vi "OlfactoryStim.vi"() -> ()   [LabVIEW 2014]
uses:
  Stim/Stim.lvclass
  <vilib>/Platform/TimedLoop/XDataNode/timing_clust.ctl
  <vilib>/Platform/TimedLoop/XDataNode/nitl_modes.ctl
  <vilib>/Platform/TimedLoop/XDataNode/wakeup.ctl
  Acquisition/Acquisition.lvclass
  <vilib>/platform/TimedLoop/XDataNode/XDataNode.xnode
  <vilib>/Platform/TimedLoop/XDataNode/XDNodeRunTimeDep.lvlib
panel:
  in  "ITA \nchannel":dbl
  in  "Cardname":string="DevOlf"
  in  "depth(um)":dbl
  in  "notes":string
  in  "filename":string
  out "error out":errorcluster
  in  "Idx":dbl[](array[numeric])
  in  "Stimulus Description":string[](array[string])
  in  "mouse_id":dbl
  out "Trial":dbl
  out "stim queue":i32
  in  "semicolon seperated stimuli":string
  in  "ITI (ms)":dbl=4000.0
  in  "Pulse Dur (ms)":dbl=4000.0
  in  "stop":bool
  out "Stim":bool[](array[boolean])
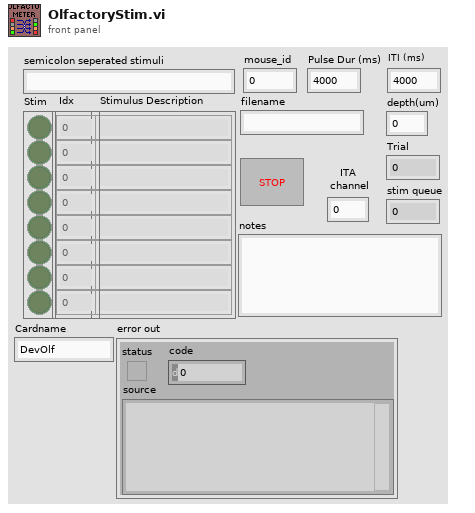
[diagram p1: front panel]
types:
  T1 = typedef "XDNodeRunTimeDep.lvlib/timing_clust.ctl" = cluster{"Expected End [f-1]":u64, "Actual End [f-1]":u64, "Finished Late? [f-1]":bool, "Expected End [i-1]":u64, "Actual End [i-1]":u64, "Finished Late? [i-1]":bool, "Expected Start [i]":u64, "Actual Start [i]":u64, "Expected Start [f]":u64, "Actual Start [f]":u64, "Source Name":string, "Structure Name":string, "Period":i64, "Deadline":i64, "Offset":i64, "Start":i64, "Priority":i32, "Timeout":i32, "Mode":T2, "Wakeup Reason":T3, "Error":errorcluster, "Source Type":string, "Secondary Source Type":string, "Global End Time":u64, "Global Start Time":u64, "Frame Duration":u64, "Iteration Duration":u64, "Assigned CPU":i32, "I/O Scan Engine Mode":u32}
  T2 = typedef "XDNodeRunTimeDep.lvlib/nitl_modes.ctl" = enum32{"No Change", "Process missed periods, maintain original phase", "Discard missed periods, maintain original phase", "Process missed periods, ignore original phase", "Discard missed periods, ignore original phase"}
  T3 = typedef "XDNodeRunTimeDep.lvlib/wakeup.ctl" = enum32{"Normal", "Aborted", "Asynchronous wakeup", "Timing source error", "Timed loop error", "Timeout"}
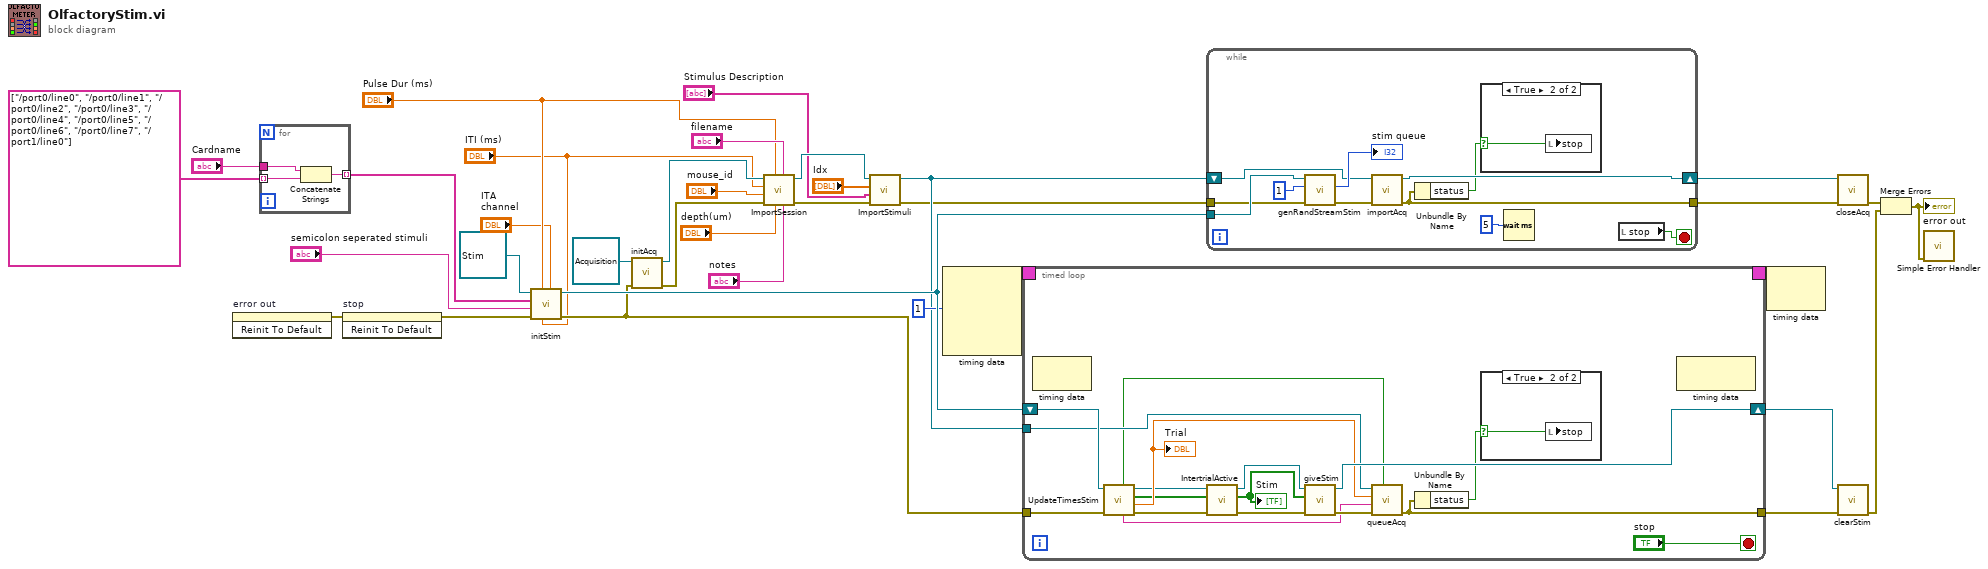
[diagram p0: block diagram]
diagram:
  n1 = invoke on="error out" class="Clust (strict)" method="Reinit To Default"() -> (error out=w17:errorcluster)  [unwired: 3 in, 2 out]
  n2 = for {
    tunnel: string[] ["/port0/line0", "/port0/line1", "/port0/line2", "/port0/line3", "/port0/line4", "/port0/line5", "/port0/line6", "/port0/line7", "/port1/line0"] ("Lines") -> [w38] mode=indexing
    tunnel: [w37] -> w6 mode=indexing
    tunnel: "Cardname" -> [w36]
    n3 = Concatenate Strings(w36, w38) -> (w37:string)
  }
  n4 = invoke on="stop" class="Bool (strict)" method="Reinit To Default"(error in=w17) -> (error out=w34:errorcluster)  [unwired: 2 in, 2 out]
  n5 = call-dynamic "initStim.vi"("ITA channel"="ITA \nchannel", "ITI"="ITI (ms)", "Pulse Duration"="Pulse Dur (ms)", "error in (no error)"=w34, "semicolon seperated stimuli"="semicolon seperated stimuli", "Lines"=w6, "Stim in"=refnum<class "Stim.lvclass"> refnum ("Stim.lvclass")) -> ("error out"=w25:errorcluster, "Stim out"=w33:refnum<class "Stim.lvclass">)  [unwired: 3 in]
  n6 = call-dynamic "initAcq.vi"("error in (no error)"=w25, "Acquisition in"=refnum<class "Acquisition.lvclass"> refnum ("Acquisition.lvclass")) -> ("error out"=w23:errorcluster, "Acquisition out"=w24:refnum<class "Acquisition.lvclass">)  [unwired: 8 in]
  n7 = call-dynamic "ImportSession.vi"("notes"="notes", "file_name"="filename", "depth"="depth(um)", "pulse_duration"="Pulse Dur (ms)", "error in (no error)"=w23, "mouse_id"="mouse_id", "intertrial_interval"="ITI (ms)", "Acquisition in"=w24) -> ("error out"=w15:errorcluster, "Acquisition out"=w16:refnum<class "Acquisition.lvclass">)  [unwired: 2 in]
  n8 = call-dynamic "ImportStimuli.vi"("error in (no error)"=w15, "stimulus Description"="Stimulus Description", "stim_idx"="Idx", "Acquisition in"=w16) -> ("error out"=w11:errorcluster, "Acquisition out"=w12:refnum<class "Acquisition.lvclass">)  [unwired: 6 in]
  n9 = node-c288(i64 1 ("Period")) -> (w29:T1)  [unwired: 3 in]
  n10 = timed-loop {
    tunnel: w25 -> [w53]
    tunnel: [w46] -> w30
    shift-right: [w55] -> w31
    shift-left: w33 -> [w54]
    timing: w29 -> [_]
    timing-out: [_] -> w28
    tunnel: w12 -> [w51]
    stop <- "stop" stop-if-true
    n11 = node-c288() -> ()  [unwired: 1 in, 1 out]
    n12 = call-dynamic "UpdateTimesStim.vi"("error in (no error)"=w53, "Stim in"=w54) -> ("error out"=w44:errorcluster, "Trial"=w49:dbl, "Juice"=w39:bool[], "Stim out"=w43:refnum<class "Stim.lvclass">, "Stimulus"=w48:string, "New trial"=w47:bool)  [unwired: 4 in]
    "Trial" <- w49
    n13 = call-dynamic "IntertrialActive.vi"("error in (no error)"=w44, "StimIn"=w39, "Stim in"=w43) -> ("error out"=w41:errorcluster, "StimOut"=w40:bool[], "Stim out"=w42:refnum<class "Stim.lvclass">)  [unwired: 6 in]
    "Stim" <- w40
    n14 = call-dynamic "giveStim.vi"("error in (no error)"=w41, "data"=w40, "Stim in"=w42) -> ("error out"=w50:errorcluster, "Stim out"=w55:refnum<class "Stim.lvclass">)  [unwired: 7 in]
    n15 = call-dynamic "queueAcq.vi"("New trial"=w47, "error in (no error)"=w50, "stimulus"=w48, "trial"=w49, "Acquisition in"=w51) -> ("error out"=w46:errorcluster)  [unwired: 4 in, 2 out]
    n16 = Unbundle By Name(w46) -> ("status"=w45:bool)
    n17 = case shown="True" w45 {
      selector: w45 -> [_ w56]
      frame False {
      }
      frame True {
        n18 = local write "stop"(w56) -> ()
      }
    }
    n19 = node-c288() -> ()  [unwired: 1 in, 1 out]
  }
  n20 = while {
    tunnel: w33 -> [w69]
    tunnel: w11 -> [w68]
    tunnel: [w60] -> w20
    shift-right: [w61] -> w21
    shift-left: w12 -> [w62]
    stop <- w64 stop-if-true
    n21 = call-dynamic "genRandStreamStim.vi"("error in (no error)"=w68, "Queue length trigger"=1, "Stim in"=w69) -> ("error out"=w63:errorcluster, "# elements in queue"=→"stim queue":i32)  [unwired: 6 in, 1 out]
    n22 = call-dynamic "importAcq.vi"("error in (no error)"=w63, "Acquisition in"=w62) -> ("error out"=w60:errorcluster, "Acquisition out"=w61:refnum<class "Acquisition.lvclass">)  [unwired: 7 in, 1 out]
    n23 = Unbundle By Name(w60) -> ("status"=w59:bool)
    n24 = case shown="True" w59 {
      selector: w59 -> [_ w70]
      frame False {
      }
      frame True {
        n25 = local write "stop"(w70) -> ()
      }
    }
    n26 = Wait (ms)(milliseconds to wait=u32 5) -> ()  [unwired: 1 out]
    n27 = local read "stop"() -> (w64:bool)
  }
  n28 = node-c288(w28) -> ()  [unwired: 1 out]
  n29 = call-dynamic "closeAcq.vi"("error in (no error)"=w20, "Acquisition in"=w21) -> ("error out"=w19:errorcluster)  [unwired: 8 in, 1 out]
  n30 = call-dynamic "clearStim.vi"("error in (no error)"=w30, "Stim in"=w31) -> ("error out"=w18:errorcluster)  [unwired: 8 in, 1 out]
  n31 = Merge Errors(w19, w18) -> (w4:errorcluster)
  "error out" <- w4
  n32 = call <vilib>:"Simple Error Handler.vi"("error in (no error)"=w4) -> ()  [unwired: 4 in, 5 out]
